vi "Format Year-Month to String.vi"(9 "Month":T1, 11 "YYYY":i32) -> (2 "Year-Mo":string)   [LabVIEW 2018]
uses:
  controls/Month.ctl
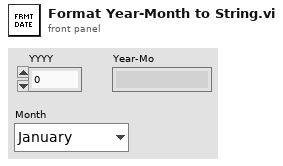
[diagram p1: front panel]
types:
  T1 = typedef "Month.ctl" = enum16{"January", "February", "March", "April", "May", "June", "July", "August", "September", "October", "November", "December"}
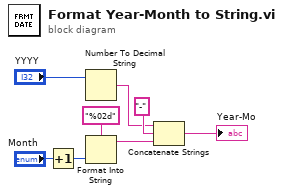
[diagram p0: block diagram]
diagram:
  n1 = Increment(x="Month") -> (x+1=w1:T1)
  n2 = Number To Decimal String(number="YYYY") -> (decimal integer string=w3:string)  [unwired: 1 in]
  n3 = Format Into String(format string="%02d" ("string"), w1) -> (resulting string=w5:string)  [unwired: 2 in, 1 out]
  n4 = Concatenate Strings(w3, "-" ("string"), w5) -> (→"Year-Mo":string)
